vi "map Modbus channels.vi"(8 "error in (no error)":errorcluster, 10 "mapping":i32, 11 "Modbus Slave configuration in":refnum<class "Modbus Slave configuration.lvclass">) -> (0 "error out":errorcluster, 3 "Modbus Slave configuration out":refnum<class "Modbus Slave configuration.lvclass">)   [LabVIEW 2013, in "Modbus Slave configuration.lvclass"]
uses:
  Modbus Slave configuration.lvclass
  Modbus Slave configuration.lvclass/Modbus Slave configuration.ctl
  module channel/Modbus Module Channel.lvclass/Modbus Module Channel.ctl
  <vilib>/NI/Tag Bus/tag/tag descriptor.lvclass/tag descriptor.ctl
  module channel/Read modbus type.vi
  <vilib>/NI/Tag Bus/tag/read data type.vi
  module channel/Write starting address.vi
  module channel/Write subindex (bool).vi
  Read modbus channels.vi
  module channel/Modbus Module Channel.lvclass
panel:
  # "0 - Custom (User Defined)\n1 - Optimized"
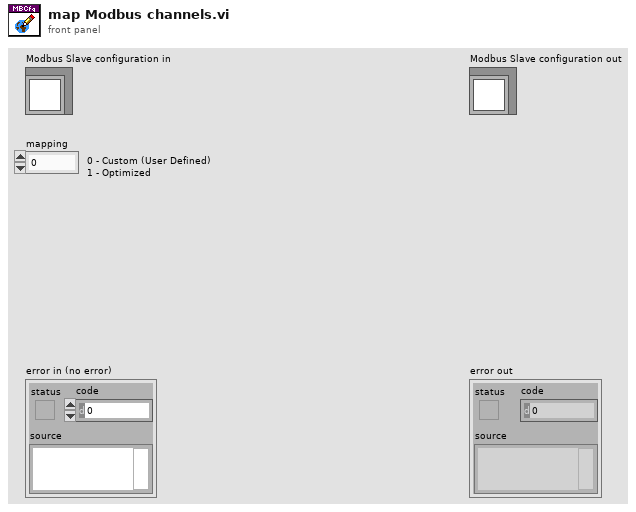
[diagram p1: front panel]
types:
  T1 = cluster{"starting address":u16, "subindex (bool)":i32}
  T2 = cluster{"starting address":u16, "subindex (bool)":i32}[]
  T3 = typedef "Modbus Module Channel.lvclass/data bank type.ctl" = enum16{"coils", "discrete inputs", "input registers", "holding registers"}
  T4 = typedef "tag bus.lvlib/tag descriptor.lvclass/Data Type.ctl" = enum16{"Double", "Single", "I64", "I32", "I16", "I8", "U64", "U32", "U16", "U8", "Boolean", "String", "Array of Double", "Array of Single", "Array of I64", "Array of I32", "Array of I16", "Array of I8", "Array of U64", "Array of U32", "Array of U16", "Array of U8", "Array of Boolean", "Array of String"}
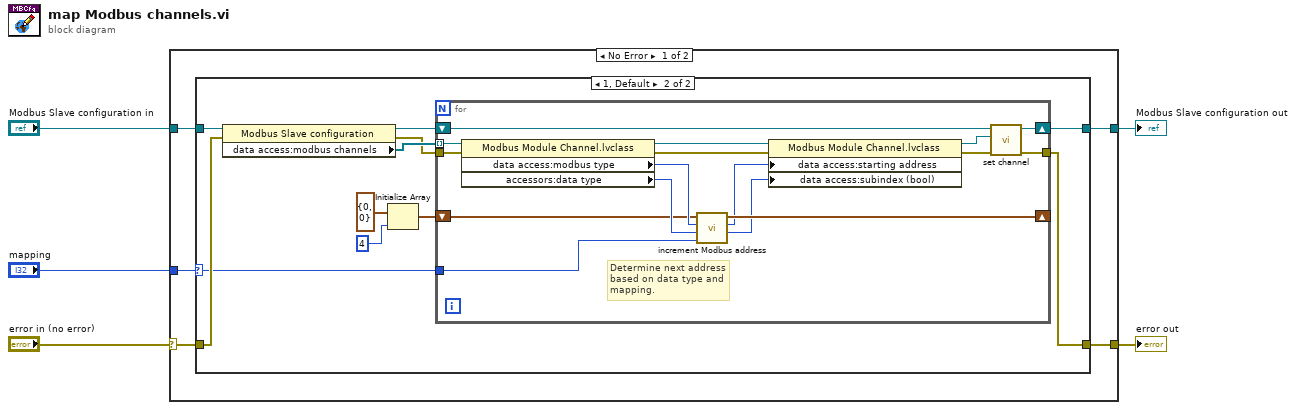
[diagram p0: block diagram]
diagram:
  n1 = case shown="No Error" "error in (no error)" {
    selector: "error in (no error)" -> [w10 w41]
    tunnel: [w7 w41] -> w4
    tunnel: [w8 w40] -> w2
    tunnel: "Modbus Slave configuration in" -> [w9 w40]
    tunnel: "mapping" -> [w6 _]
    frame No Error {
      n2 = case shown="1, Default" w6 {
        selector: w6 -> [_ w13]
        tunnel: w10 -> [w11 w22]
        tunnel: w9 -> [w12 w21]
        tunnel: [w12 w16] -> w8
        tunnel: [w11 w14] -> w7
        frame 0 {
          # "Custom mapping (User Defined), \nso the configuration is left\nunchanged."
        }
        frame 1, Default {
          n3 = property class="Modbus Slave configuration"(reference=w21, error in=w22) -> (reference out=w17:refnum<class "Modbus Slave configuration.lvclass">, error out=w15:errorcluster, "data access:modbus channels"=w23:refnum<class "Modbus Module Channel.lvclass">[])
          n4 = Initialize Array(T1 {"starting address"=0, "subindex (bool)"=0} ("next open address"), 4 ("dimension size")) -> (w18:T2)
          n5 = for {
            tunnel: w23 -> [w39] mode=indexing
            shift-right: [w26] -> _
            shift-left: w18 -> [w28]
            tunnel: w13 -> [w27]
            shift-right: [w35] -> w16
            shift-left: w17 -> [w36]
            tunnel: w15 -> [w34]
            tunnel: [w31] -> w14
            # "Determine next address \nbased on data type and \nmapping."
            n6 = property class="Modbus Module Channel.lvclass"(reference=w39, error in=w34) -> (reference out=w38:refnum<class "Modbus Module Channel.lvclass">, error out=w33:errorcluster, "data access:modbus type"=w29:T3, "accessors:data type"=w30:T4)
            n7 = call "increment Modbus address.vi"("mapping"=w27, "data type"=w30, "modbus type"=w29, "available addresses"=w28) -> ("subindex (bool)"=w24:i32, "starting address"=w25:u16, "available addresses out"=w26:T2)  [unwired: 5 in]
            n8 = property class="Modbus Module Channel.lvclass"(reference=w38, error in=w33, "data access:starting address"=w25, "data access:subindex (bool)"=w24) -> (reference out=w37:refnum<class "Modbus Module Channel.lvclass">, error out=w32:errorcluster)
            n9 = call "set channel.vi"("error in"=w32, "Modbus Module Channel.lvclass"=w37, "Modbus Slave configuration in"=w36) -> ("error out"=w31:errorcluster, "Modbus Slave configuration out"=w35:refnum<class "Modbus Slave configuration.lvclass">)  [unwired: 7 in]
          }
        }
      }
    }
    frame Error {
    }
  }
  "error out" <- w4
  "Modbus Slave configuration out" <- w2
